vi "03 - Staged create-verify-staged update-archive.vi"   [LabVIEW 2020]
uses:
  client/client.lvlib
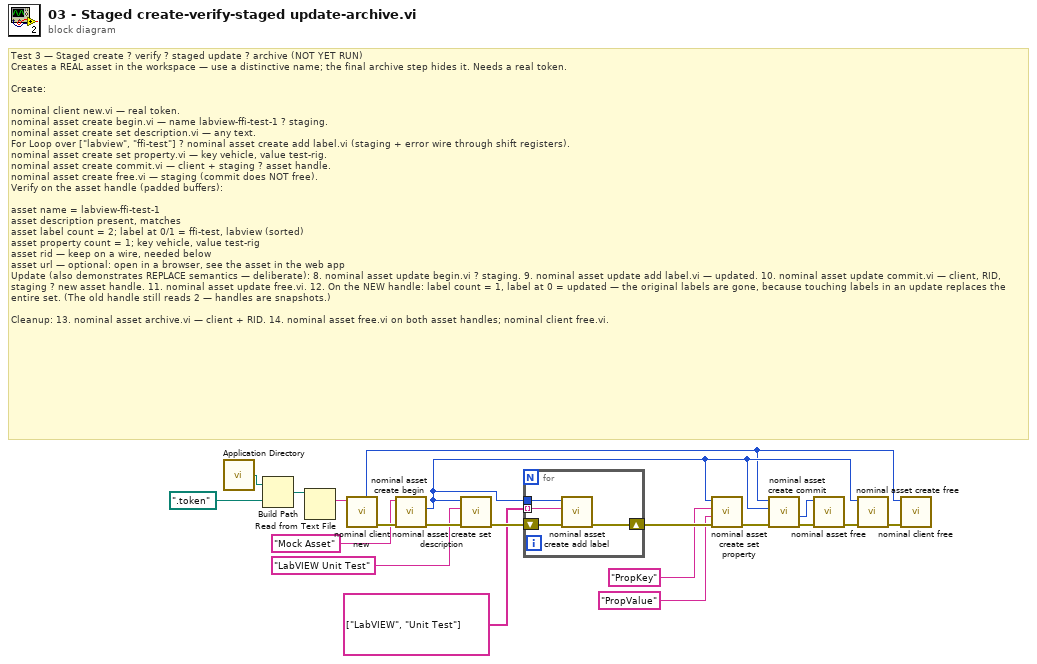
[diagram p0: block diagram]
diagram:
  # "Test 3 — Staged create ? verify ? staged update ? archive (NOT YET RUN)\nCreates a REAL asset in the workspace — use a distinctive name; the final archive step hides it. Needs a real token.\n\nCreate:\n\nnominal client new.vi — real token.\nnominal asset create begin.vi — name labview-ffi-test-1 ? staging.\nnominal asset create set description.vi — any text.\nFor Loop over [\"labview\", \"ffi-test\"] ? nominal asset create add label.vi (staging + error wire through shift registers).\nnominal asset create set property.vi — key vehicle, value test-rig.\nnominal asset create commit.vi — client + staging ? asset handle.\nnominal asset create free.vi — staging (commit does NOT free).\nVerify on the asset handle (padded buffers):\n\nasset name = labview-ffi-test-1\nasset description present, matches\nasset label count = 2; label at 0/1 = ffi-test, labview (sorted)\nasset property count = 1; key vehicle, value test-rig\nasset rid — keep on a wire, needed below\nasset url — optional: open in a browser, see the asset in the web app\nUpdate (also demonstrates REPLACE semantics — deliberate): 8. nominal asset update begin.vi ? staging. 9. nominal asset update add label.vi — updated. 10. nominal asset update commit.vi — client, RID, staging ? new asset handle. 11. nominal asset update free.vi. 12. On the NEW handle: label count = 1, label at 0 = updated — the original labels are gone, because touching labels in an update replaces the entire set. (The old handle still reads 2 — handles are snapshots.)\n\nCleanup: 13. nominal asset archive.vi — client + RID. 14. nominal asset free.vi on both asset handles; nominal client free.vi."
  n1 = call <vilib>:"Application Directory.vi"() -> ("Application Directory"=w10:path)
  n2 = Build Path(base path=w10, name or relative path=path ".token") -> (appended path=w8:path)
  n3 = Read from Text File(file (use dialog)=w8) -> (text=w7:string)  [unwired: 3 in, 3 out]
  n4 = call "nominal client new.vi"("token"=w7) -> ("error out"=w20:errorcluster, "out_client out"=w12:i32)  [unwired: 8 in, 1 out]
  n5 = call "nominal asset create begin.vi"("error in (no error)"=w20, "name"="Mock Asset") -> ("error out"=w19:errorcluster, "out_staging out"=w14:i32)  [unwired: 7 in, 1 out]
  n6 = call "nominal asset create set description.vi"("error in (no error)"=w19, "description"="LabVIEW Unit Test", "staging"=w14) -> ("error out"=w18:errorcluster)  [unwired: 7 in, 1 out]
  n7 = for {
    tunnel: w14 -> [w24]
    shift-right: [w22] -> w17
    shift-left: w18 -> [w23]
    tunnel: string[] ["LabVIEW", "Unit Test"] ("label") -> [w21] mode=indexing
    n8 = call "nominal asset create add label.vi"("error in (no error)"=w23, "label"=w21, "staging"=w24) -> ("error out"=w22:errorcluster)  [unwired: 7 in, 1 out]
  }
  n9 = call "nominal asset create set property.vi"("error in (no error)"=w17, "value"="PropValue" ("key"), "key"="PropKey", "staging"=w14) -> ("error out"=w16:errorcluster)  [unwired: 6 in, 1 out]
  n10 = call "nominal asset create commit.vi"("error in (no error)"=w16, "staging"=w14, "client"=w12) -> ("error out"=w2:errorcluster, "out_asset out"=w3:i32)  [unwired: 6 in, 1 out]
  n11 = call "nominal asset free.vi"("error in (no error)"=w2, "asset"=w3) -> ("error out"=w1:errorcluster)  [unwired: 8 in, 1 out]
  n12 = call "nominal asset create free.vi"("error in (no error)"=w1, "staging"=w14) -> ("error out"=w15:errorcluster)  [unwired: 8 in, 1 out]
  n13 = call "nominal client free.vi"("error in (no error)"=w15, "client"=w12) -> ()  [unwired: 8 in, 2 out]
